vi "Write Socket Config.vi"(8 "error in (no error)":errorcluster, 10 "Socket Config":T1={"Socket type"=enum."ZMQ_PUB", "endpoint"="tcp://*:5555", "socket filter"=""}, 11 "0MQ_Server in":refnum<class "0MQ_Server.lvclass">) -> (0 "error out":errorcluster, 3 "0MQ_Server out":refnum<class "0MQ_Server.lvclass">)   [LabVIEW 2016, in "0MQ_Server.lvclass"]
uses:
  0MQ_Server.lvclass
  Typedefs/Socket Config.ctl
  <vilib>/addons/zeromq/socket_type.ctl
  0MQ_Server.lvclass/0MQ_Server.ctl
  <vilib>/addons/zeromq/zeromq.lvlib
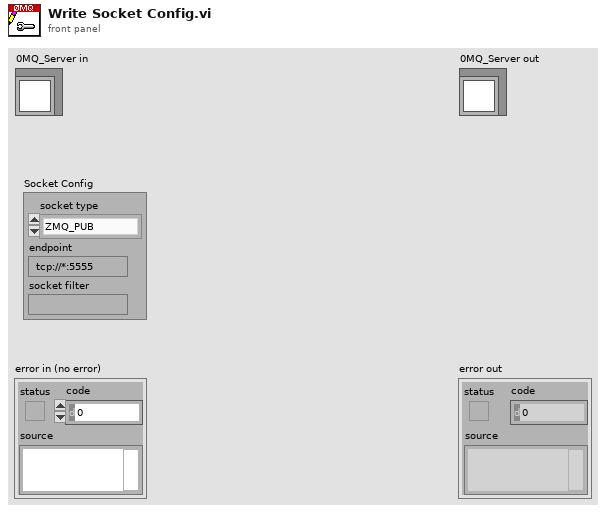
[diagram p1: front panel]
types:
  T1 = typedef "0MQ_Server.lvclass/Socket Config.ctl" = cluster{"Socket type":T2, "endpoint":string, "socket filter":string}
  T2 = typedef "zeromq.lvlib/socket_type.ctl" = enum8{"ZMQ_PAIR", "ZMQ_PUB", "ZMQ_SUB", "ZMQ_REQ", "ZMQ_REP", "ZMQ_DEALER", "ZMQ_ROUTER", "ZMQ_PULL", "ZMQ_PUSH", "ZMQ_XPUB", "ZMQ_XSUB"}
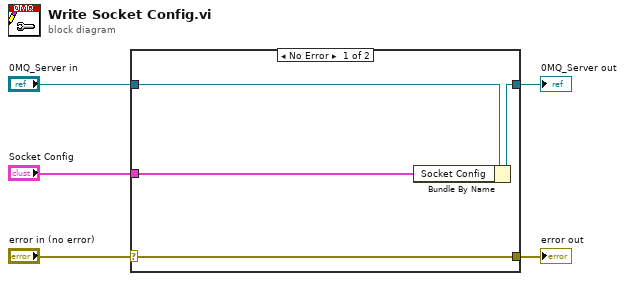
[diagram p0: block diagram]
diagram:
  n1 = case shown="No Error" "error in (no error)" {
    selector: "error in (no error)" -> [w9 w10]
    tunnel: [w9 w10] -> w4
    tunnel: [w7 w11] -> w2
    tunnel: "0MQ_Server in" -> [w8 w11]
    tunnel: "Socket Config" -> [w6 _]
    frame No Error {
      n2 = Bundle By Name(cluster=w8, "Socket Config"=w6) -> (w7:refnum<class "0MQ_Server.lvclass">)
    }
    frame Error {
    }
  }
  "error out" <- w4
  "0MQ_Server out" <- w2
